vi "UHR-Fleezers Control (host) - Lorentz v4.vi"() -> ()   [LabVIEW 2014] (continued)
        n901 = case shown="True" w1439 {
          tunnel: w1436 -> [_ w1446]
          frame False {
          }
          frame True {
            n902 = local read "Time (s)"() -> (w1447:dbl)
            n903 = local read "log file ref"() -> (w1448:refnum<file>)
            n904 = call "write to event log.vi"("log file ref"=w1448, "time"=w1447, "input string"=w1446) -> ()  [unwired: 8 in]
          }
        }
        n905 = call "preamp serial write macro.vi"("String"=w1441, "Delay (ms)"=w1442, "VISA resource name"=w1445) -> ("read buffer"=→"Reply":string, "error out"=w1444:errorcluster)  [unwired: 1 out]
        n906 = call "preamp serial write macro.vi"("String"=w1441, "Delay (ms)"=w1442, "VISA resource name"=w1440) -> ()  [unwired: 3 out]
        n907 = local write "Preamp Error Out"(w1444) -> ()
      }
    }
    n908 = node-c288() -> ()  [unwired: 1 in, 1 out]
  }
  n909 = flat-sequence "Safety limits on RF frequencies and amplitudes (for AOM protection)" {
    tunnel: [w1527] -> w38
    tunnel: [w1525] -> w40
    tunnel: [w1528] -> w41
    tunnel: [w1529] -> w39
    tunnel: w22 -> [w1527]
    tunnel: T24 {"Minimum"=0.0, "Maximum"=50.0, "Increment"=1.0} ("Data Entry Limits") -> [w1525]
    tunnel: w27 -> [w1526]
    tunnel: [w1526] -> w42
    frame #0 {
      w1529 = T24 {"Minimum"=0.0, "Maximum"=40.0, "Increment"=0.1} ("Min Max Inc")
      w1528 = T24 {"Minimum"=0.0, "Maximum"=45.0, "Increment"=1.0} ("Data Entry Limits")
      n910 = property on="BD 2 Frequency 1 (MHz)" class="DigNum (strict)"("Data Range"=w1529) -> ()  [unwired: 2 in, 2 out]
      n911 = property on="BD 2 Frequency 3 (MHz)" class="DigNum (strict)"("Data Range"=w1529) -> ()  [unwired: 2 in, 2 out]
      n912 = property on="BD 2 Frequency 2 (MHz)" class="DigNum (strict)"("Data Range"=w1529) -> ()  [unwired: 2 in, 2 out]
      n913 = property on="BD 1 Frequency 1 (MHz)" class="DigNum (strict)"("Data Range"=w1527) -> ()  [unwired: 2 in, 2 out]
      n914 = property on="BD 1 Frequency 2 (MHz)" class="DigNum (strict)"("Data Range"=w1527) -> ()  [unwired: 2 in, 2 out]
      n915 = property on="BD 1 Frequency 3 (MHz)" class="DigNum (strict)"("Data Range"=w1527) -> ()  [unwired: 2 in, 2 out]
      n916 = property on="BD 2 Amplitude 1 (%)" class="DigNum (strict)"("Data Range"=w1528) -> ()  [unwired: 2 in, 2 out]
      n917 = property on="BD 2 Amplitude 2 (%)" class="DigNum (strict)"("Data Range"=w1528) -> ()  [unwired: 2 in, 2 out]
      n918 = property on="BD 2 Amplitude 3 (%)" class="DigNum (strict)"("Data Range"=w1528) -> ()  [unwired: 2 in, 2 out]
      n919 = property on="BD 1 Amplitude 3 (%)" class="DigNum (strict)"("Data Range"=w1525) -> ()  [unwired: 2 in, 2 out]
      n920 = property on="BD 1 Amplitude 2 (%)" class="DigNum (strict)"("Data Range"=w1525) -> ()  [unwired: 2 in, 2 out]
      n921 = property on="BD 1 Amplitude 1 (%)" class="DigNum (strict)"("Data Range"=w1525) -> ()  [unwired: 2 in, 2 out]
      "X RF Frequency Limits (MHz)" <- w1527
      "X RF Amplitude Limits (%)" <- w1525
      "Y RF Amplitude Limits (%)" <- w1528
      "Y RF Frequency Limits (MHz)" <- w1529
    }
  }
  n922 = stacked-sequence "Host initialization sequence - order matters!" {
    tunnel: w42 -> [_ w1549 w1641 _ w1698 w1707 w1774 w1798 _ w1841 _]
    tunnel: [_ _ _ _ _ _ _ _ _ w1841 _] -> w31
    tunnel: [_ _ _ _ _ _ _ _ _ w1840 _] -> w44
    tunnel: w41 -> [_ _ _ _ _ _ w1772 _ _ _ _]
    tunnel: w40 -> [_ _ _ _ _ _ w1771 _ _ _ _]
    tunnel: w39 -> [_ _ _ _ _ _ w1770 _ _ _ _]
    tunnel: w38 -> [_ _ _ _ _ _ w1751 _ _ _ _]
    tunnel: [_ _ _ _ _ _ _ _ w1838 _ _] -> _
    tunnel: [_ _ _ _ _ _ _ _ _ _ w1842] -> w21
    tunnel: [_ _ _ _ _ _ _ _ _ _ w1843] -> w20
    frame #0 {
    }
    frame #1 {
      w1581 = 10.0 ("y")
      w1582 = 32767.0 ("y")
      w1566 = 6.0  # clock mult.
      w1565 = 49152000.0  # TCXO frequ.
      # "Initialize some FPGA settings"
      n923 = local read "Not-Interlacing Set"() -> (w1621:enum32{"Set 1", "Set 2", "Set 3"})
      n924 = local write "Trap Pos FIFO Timeout"(u16 0 ("Trap Pos FIFO Timeout")) -> ()
      n925 = local read "Interlace"() -> (w1619:bool)
      n926 = local read "Desired Scan Incr (V)"() -> (w1593:dbl)
      n927 = local read "BD 1 Delay (ticks)"() -> (w1628:u8)
      n928 = local read "Number Interlace Sets"() -> (w1620:u8)
      n929 = local read "BD 2 Delay (Ticks)"() -> (w1629:u8)
      n930 = property on="AI Count (ticks)" class="DigNum (strict)"("Val(Sgnl)"="AI Count (ticks)") -> ()  [unwired: 2 in, 2 out]
      n931 = local read "AO1"() -> (w1587:dbl)
      n932 = local read "AO2"() -> (w1588:dbl)
      n933 = local read "Next trap write delay (ticks)"() -> (w1630:u8)
      n934 = local read "Number of scans (MCL)"() -> (w1597:u64)
      n935 = local read "Cycles/step (MCL)"() -> (w1596:u64)
      n936 = local read "Scan steps (MCL)"() -> (w1595:u64)
      n937 = local read "Continuous MCL Scanning"() -> (w1598:bool)
      n938 = Multiply(x=w1587, y=w1582) -> (x*y=w1585:dbl)
      n939 = Multiply(x=w1588, y=w1582) -> (x*y=w1583:dbl)
      n940 = Build Array("DIO count 1 (ticks)", "DIO count 2 (ticks)", "DIO count 3 (ticks)") -> (w1614:u16[])
      n941 = local read "Fast Scan Dir"() -> (w1599:bool)
      n942 = local read "2D or 1D Scan"() -> (w1611:bool)
      n943 = local read "N Acq Sets (Traps + Fl.)"() -> (w1607:i16)
      n944 = local read "Scan Increment (MHz)"() -> (w1570:dbl)
      n945 = Divide(x=w1585, y=w1581) -> (x/y=w1586:dbl)
      n946 = Divide(x=w1583, y=w1581) -> (x/y=w1584:dbl)
      n947 = To Unsigned Byte Integer(number=w1621) -> (unsigned 8bit integer=w1616:u8)
      n948 = Split 1D Array(array=w1614, index=w1620) -> (first subarray=w1612:u16[])  [unwired: 1 out]
      n949 = Multiply(x=w1593, y=32767.0) -> (x*y=w1591:dbl)
      n950 = To Word Integer(number=w1586) -> (16bit integer=w1532:i16)
      n951 = To Word Integer(number=w1584) -> (16bit integer=w1531:i16)
      n952 = Index Array(array=w1614, index=w1616) -> (element=w1615:u16)
      n953 = Add Array Elements(numeric array=w1612) -> (sum=w1613:u16)
      n954 = Multiply(x=w1565, y=w1566) -> (x*y=w1567:dbl)
      n955 = Divide(x=w1591, y=10.0) -> (x/y=w1592:dbl)
      n956 = Select(t=w1613, s=w1619, f=w1615) -> (s? t:f=w1622:u16)
      n957 = Not(x=w1599) -> (.not. x?=w1600:bool)
      n958 = To Word Integer(number=w1592) -> (16bit integer=w1594:i16)
      n959 = property on="2D or 1D Scan" class="Bool (strict)"("Val(Sgnl)"=w1611) -> ()  [unwired: 2 in, 2 out]
      n960 = Divide(x=40000000.0, y="AI Count (ticks)") -> (x/y=w1603:dbl)
      n961 = local write "Update Count (MCL)"(w1622) -> ()
      n962 = local write "Total Counts (ticks)"(w1622) -> ()
      n963 = Divide(x=w1603, y="FPGA Ave.") -> (x/y=w1602:dbl)
      n964 = local write "AI rate (Hz)"(w1603) -> ()
      n965 = Multiply(x=w1570, y=1000.0) -> (x*y=w1563:dbl)
      n966 = local write "Ave. Rate (Hz)"(w1602) -> ()
      n967 = Reciprocal(x=w1602) -> (1/x=w1601:dbl)
      n968 = Scale By Power Of 2(n=48, x=w1563) -> (x*2^n=w1562:dbl)
      n969 = local write "Ave. Period (s)"(w1601) -> ()
      n970 = Divide(x=w1562, y=w1567) -> (x/y=w1568:dbl)
      n971 = To Quad Integer(1:w1568) -> (0:w1571:i64)
      n972 = local read "Setpoints (V)"() -> (w1556:cluster{"Set 1":dbl, "Set 2":dbl})
      n973 = local read "# Samples/channel"() -> (w1578:u32)
      n974 = local read "Feedback On/Off"() -> (w1553:cluster{"Set 1":bool, "Set 2":bool})
      n975 = local read "T3 Y (V)"() -> (w1536:dbl)
      n976 = local read "T3 X (V)"() -> (w1535:dbl)
      n977 = local read "Trap intensity output range"() -> (w1546:cluster{"Normal High":i16, "Normal Low":i16})
      n978 = local read "All FB On/Off"() -> (w1552:bool)
      n979 = local read "Number of F/B Scans (AOD)"() -> (w1577:u16)
      n980 = local read "Trap Intensity PID Gains"() -> (w1545:T14)
      n981 = local read "Cycles/step (AOD)"() -> (w1573:u64)
      n982 = local read "Scan steps (AOD)"() -> (w1572:u64)
      n983 = Multiply(x=w1572, y=w1573) -> (x*y=w1574:u64)
      n984 = Multiply(x=w1574, y=u64 2) -> (x*y=w1576:u64)
      n985 = Multiply(x=w1576, y=w1577) -> (x*y=w1579:u64)
      n986 = Multiply(x=3276.7, y=w1556) -> (x*y=w1557:cluster{"Set 1":dbl, "Set 2":dbl})
      n987 = local read "Scan BD"() -> (w1561:bool)
      n988 = Multiply(x=w1536, y=32767.0) -> (x*y=w1542:dbl)
      n989 = And(x=w1553, y=w1552) -> (x .and. y?=w1554:cluster{"Set 1":bool, "Set 2":bool})
      n990 = To Word Integer(number=w1557) -> (16bit integer=w1558:cluster{"Set 1":i16, "Set 2":i16})
      n991 = Multiply(x=w1535, y=32767.0) -> (x*y=w1539:dbl)
      n992 = local read "Sets to FIFO (Traps)"() -> (w1624:T22)
      n993 = Divide(x=w1579, y=w1578) -> (x/y=w1580:dbl)
      n994 = Unbundle By Name(w1554) -> ("Set 1"=w1550:bool, "Set 2"=w1551:bool)
      n995 = Unbundle By Name(w1558) -> ("Set 1"=w1559:i16, "Set 2"=w1560:i16)
      n996 = Divide(x=w1542, y=10.0) -> (x/y=w1543:dbl)
      n997 = Divide(x=w1539, y=10.0) -> (x/y=w1538:dbl)
      n998 = To Unsigned Word Integer(number=w1543) -> (unsigned 16bit integer=w1534:u16)
      n999 = To Unsigned Word Integer(number=w1538) -> (unsigned 16bit integer=w1533:u16)
      n1000 = local read "FPGA error out"() -> (w1548:errorcluster)
      n1001 = local write "Data points/scan (f/b)"(w1576) -> ()
      n1002 = local write "Data points/scans"(w1579) -> ()
      n1003 = local write "N sets should be saved"(w1580) -> ()
      n1004 = Unbundle By Name(w1624) -> ("Set 1"=w1625:bool, "Set 2"=w1626:bool, "Set 3"=w1627:bool)
      n1005 = xnode "Read/Write Control"("FPGA VI Reference In"=w1549, "error in"=w1548, "ai count"="AI Count (ticks)", "Interlace ON/OFF"=w1619, "Number Interlace Cycles"=w1620, "Set 1"=w1625, "Set 2"=w1626, "Set 3"=w1627, "FB On/Off Set 1"=w1550, "FB On/Off Set 2"=w1551, "Interlace Off Parameters"=w1621, "FB Setpoint Set 1"=w1559, "FB Setpoint Set 2"=w1560, "Piezo Trap Y (AO4)"=w1534, "Piezo Trap X (AO5)"=w1533, "FB Gains"=w1545, "FB output range"=w1546, "Cycles per step"=w1573, "Scan BD"=w1561, "Number of scans"=w1577, "Scan steps"=w1572, "Scan freq.  increment"=w1571, "AO1"=w1532, "AO2"=w1531, "Scan freq.  increment (MCL)"=w1594, "Scan steps (MCL)"=w1595, "Cycles per step (MCL)"=w1596, "Number of scans (MCL)"=w1597, "MCL count"=w1622, "Cont. Scan (MCL)"=w1598, "MCL Scan Axis"=w1600, "1D or 2D Scan?"=w1611, "N of AI1 Int Acq Sets"=w1607, "Amp switch delay"="Amp switch delay", "Swap F1 and F2"="Swap F1 and F2", "APD to FIFO"=FALSE, "DIO count 1 (ticks)"="DIO count 1 (ticks)", "DIO count 2 (ticks)"="DIO count 2 (ticks)", "DIO count 3 (ticks)"="DIO count 3 (ticks)", "BD 1 Delay (ticks)"=w1628, "BD 2 Delay (Ticks)"=w1629, "Next trap write delay (ticks)"=w1630) -> ("error out"=w1547:errorcluster)  [unwired: 1 out]
      n1006 = local write "FPGA error out"(w1547) -> ()
    }
    frame #2 {
      # "Initialize some more FPGA settings"
      n1007 = local read "Trap Pos FB Monitor\nT1 or T2"() -> (w1652:bool)
      n1008 = local read "Trap Pos FB Negate Action"() -> (w1653:bool)
      n1009 = local read "Trap Pos. FB Offset Factor"() -> (w1654:i64)
      n1010 = local read "Trap Pos. FB Mult Factor"() -> (w1655:i64)
      n1011 = local read "Trap Pos. AI1 X Pre-scale"() -> (w1657:u16)
      n1012 = local read "Trap Pos FB Int Count"() -> (w1659:u16)
      n1013 = local read "Green Laser ON"() -> (w1631:bool)
      n1014 = local read "Neg. TTrig FPGA"() -> (w1660:bool)
      n1015 = local read "Trap Pos. FB Range"() -> (w1636:T18)
      n1016 = local read "Trap Pos. FB Gains"() -> (w1637:T17)
      n1017 = local read "Dynamic Force FB (ronen)"() -> (w1638:bool)
      n1018 = Multiply(x="Green Intensity % (FB OFF)", y=655.35) -> (x*y=w1646:dbl)
      n1019 = Multiply(x="Red FB Setpoint (mV)", y=3.2767) -> (x*y=w1668:dbl)
      n1020 = Multiply(x="Red Intensity % (FB OFF)", y=655.35) -> (x*y=w1672:dbl)
      n1021 = Unbundle By Name("Red FB Gains") -> ("proportional gain (Kc)"=w1677:i16, "integral gain (Kc*Ts/Ti)"=w1678:i16, "derivative gain (Kc*Td/Ts)"=w1679:i16)
      n1022 = Multiply(x="Green FB Setpoint (mV)", y=3.2767) -> (x*y=w1649:dbl)
      n1023 = To Unsigned Word Integer(number=w1646) -> (unsigned 16bit integer=w1648:u16)
      n1024 = To Unsigned Word Integer(number=w1672) -> (unsigned 16bit integer=w1675:u16)
      n1025 = To Word Integer(number=w1668) -> (16bit integer=w1671:i16)
      n1026 = local read "Differential FB?"() -> (w1662:bool)
      n1027 = To Word Integer(number=w1649) -> (16bit integer=w1651:i16)
      n1028 = local read "Laser interlacing mode"() -> (w1634:enum32{"Laser ON", "Laser OFF", "Interlace"})
      n1029 = local read "Invert laser interlacing"() -> (w1635:bool)
      n1030 = Unbundle By Name("Green FB Gains") -> ("proportional gain (Kc)"=w1665:i16, "integral gain (Kc*Ts/Ti)"=w1666:i16, "derivative gain (Kc*Td/Ts)"=w1667:i16)
      n1031 = Select(t=w1634, s=w1631, f=enum32{"Laser ON", "Laser OFF", "Interlace"}."Laser OFF" ("Green laser mode")) -> (s? t:f=w1633:enum32{"Laser ON", "Laser OFF", "Interlace"})
      n1032 = local read "FPGA error out"() -> (w1639:errorcluster)
      n1033 = xnode "Read/Write Control"("FPGA VI Reference In"=w1641, "error in"=w1639, "Invert GI"=w1635, "Invert GI 2"=w1635, "Invert RI"=w1635, "Invert RI 2"=w1635, "Operating Mode"=w1633, "Operating Mode 2"=w1633, "Red Laser Operating Mode"=w1633, "RI Operating Mode 2"=w1633, "P3"=w1665, "I3"=w1666, "D3"=w1667, "Green FB Setpoint"=w1651, "Green FB On/Off"="Green FB On/Off", "Current Out"=w1648, "Green int current ON count adj"="Green int current ON count adj", "Trap Pos FB Monitor T1 or T2"=w1652, "Trap Pos FB Negate Action"=w1653, "Trap Pos. FB Offset Factor"=w1654, "Trap Pos. FB Mult Factor"=w1655, "Force feedback"=FALSE, "AI1 X Scale"=w1657, "Trap Pos to FIFO"=TRUE, "Trap Pos FB Int Count"=w1659, "TTrig Negate Pos"=w1660, "FB Trig Integrate"="FB Trig Integrate", "Diff FB Measurement?"=w1662, "Negate Diff?"="Negate Diff?", "Trap pos. FB Range"=w1636, "Trap Pos. FB Gains"=w1637, "Red FB Setpoint"=w1671, "RI Current Out"=w1675, "P4"=w1677, "I4"=w1678, "D4"=w1679, "Red FB On/Off"="Red FB On/Off", "Dynamic Force FB (Ronen)"=w1638) -> ("error out"=w1640:errorcluster)  [unwired: 1 out]
      n1034 = local write "FPGA error out"(w1640) -> ()
    }
    frame #3 {
      # "Initialize more settings. Should stop using event loops to initialize."
      # "What are these?"
      n1035 = local write "Offset (nm)"(0.0 ("Offset (nm)")) -> ()
      n1036 = local write "Bead Mean (nm)"(0.0 ("Bead Mean (nm)")) -> ()
      n1037 = stacked-sequence {
        frame #0 {
          w1683 = T54."empty" ("mode")
          # "Clear external fluorescence triggering FIFO"
          # "APD loop counts"
          # "Fluorescence loop counts (rates)"
          n1038 = local read "APD Integration Time (s)"() -> (w1685:dbl)
          n1039 = local read "Interlace ON count"() -> (w1686:u16)
          n1040 = call "Smart Buffer (DBL) 1.vi"("mode"=w1683) -> ()  [unwired: 5 in, 6 out]
          n1041 = call "Smart Buffer (DBL) 2.vi"("mode"=w1683) -> ()  [unwired: 5 in, 6 out]
          n1042 = property on="APD Integration Time (s)" class="DigNum (strict)"("Val(Sgnl)"=w1685) -> ()  [unwired: 2 in, 2 out]
          n1043 = property on="Interlace ON count" class="DigNum (strict)"("Val(Sgnl)"=w1686) -> ()  [unwired: 2 in, 2 out]
          "Number of APDs" <- 3.0 ("Number of APDs")
        }
        frame #1 {
          # "Number of APDs affects\nAPD DMA transfer"
          # "General settings for all lasers:"
          # "And includes all laser\nON/OFF settings"
          # "Fluorescent lasers settings:"
          # "Blue laser settings:"
          n1044 = local read "Laser interlacing mode"() -> (w1688:enum32{"Laser ON", "Laser OFF", "Interlace"})
          n1045 = local read "Invert laser interlacing"() -> (w1687:bool)
          n1046 = local read "Blue FB On/Off"() -> (w1689:bool)
          n1047 = property on="Blue FB On/Off" class="Bool (strict)"("Val(Sgnl)"=w1689) -> ()  [unwired: 2 in, 2 out]
          n1048 = property on="Invert laser interlacing" class="Bool (strict)"("Val(Sgnl)"=w1687) -> ()  [unwired: 2 in, 2 out]
          n1049 = property on="Laser interlacing mode" class="RadioBtnsControl (strict)"("Val(Sgnl)"=w1688) -> ()  [unwired: 2 in, 2 out]
        }
        frame #2 {
          w1690 = path "C:/Home/Bustamante Lab/Comstock-LabView-Link.udl" ("connection information")
          # "Database link changed by Ronen - not clear if it matter for the program."
          # "Initialize the database connection"
          n1050 = disable-structure shown="Disabled" {
            disable-tunnel: [w1693 _] -> w1691
            disable-tunnel: w1690 -> [w1692 _]
            frame Disabled {
              n1051 = call-poly <vilib>:"DB Tools Open Connection.vi"("connection information"=w1692) -> ("connection reference"=w1693:T25)  [unwired: 7 in, 1 out]
            }
            frame Enabled {
            }
          }
          "connection reference" <- w1691
          n1052 = local write "connection reference"(w1691) -> ()
          n1053 = local write "Database link"(w1690) -> ()
        }
        frame #3 {
          # "Load active calibration to fpga"
          n1054 = local read "Base N trap periods"() -> (w1695:u32)
          n1055 = local read "T1 Osc Enable"() -> (w1694:bool)
          n1056 = property on="T1 Osc Enable" class="Bool (strict)"("Val(Sgnl)"=w1694) -> ()  [unwired: 2 in, 2 out]
          n1057 = property on="Base N trap periods" class="DigNum (strict)"("Val(Sgnl)"=w1695) -> ()  [unwired: 2 in, 2 out]
        }
      }
    }
    frame #4 {
      # "Set FIFO size and run FPGA"
      n1058 = local read "FPGA error out"() -> (w1697:errorcluster)
      n1059 = xnode "Invoke Method"("FPGA VI Reference In"=w1698, "error in"=w1697, "Requested Depth"="Trap AI FIFO Depth") -> ("FPGA VI Reference Out"=w1702:T50, "error out"=w1703:errorcluster)  [unwired: 1 out]
      n1060 = xnode "Invoke Method"("FPGA VI Reference In"=w1702, "error in"=w1703, "Requested Depth"="Trap Position FIFO Depth") -> ("FPGA VI Reference Out"=w1700:T50, "error out"=w1699:errorcluster)  [unwired: 1 out]
      n1061 = xnode "Invoke Method"("FPGA VI Reference In"=w1700, "error in"=w1699) -> ("error out"=w1696:errorcluster)  [unwired: 1 in, 1 out]
      n1062 = local write "FPGA error out"(w1696) -> ()
    }
    frame #5 {
      # "Adjust FPGA timing loop phases"
      n1063 = flat-sequence "Initial FPGA Loop Relative Phase Adjustment" {
        tunnel: "Initial Phase Adjustment (AI1)" -> [w1737]
        tunnel: "Initial Phase Adjustment (GI)" -> [w1736]
        tunnel: "Initial Phase Adj. (MCL)" -> [w1735]
        tunnel: [w1738] -> w1722
        tunnel: [w1734] -> w1721
        tunnel: "Initial Phase Adjustment (APD Acq)" -> [w1733]
        tunnel: "Initial Phase Adjustment (APD 1 Gate)" -> [w1732]
        tunnel: "Initial Phase Adjustment (Green FB)" -> [w1731]
        tunnel: "Initial Phase Adjustment (GI) 2" -> [w1730]
        tunnel: "Initial Phase Adjustment (APD 2 Gate)" -> [w1729]
        tunnel: "Initial Phase Adjustment (RI)" -> [w1728]
        tunnel: "Initial Phase Adjustment (BI DO)" -> [w1727]
        tunnel: "Initial Phase Adjustment (BI AO)" -> [w1726]
        tunnel: "Initial Phase Adjustment (APD 3 Gate)" -> [w1725]
        tunnel: w1707 -> [w1724]
        tunnel: w1722 -> [w1740]
        tunnel: [w1741] -> w1720
        tunnel: w1721 -> [w1741]
        tunnel: [w1740] -> w1719
        tunnel: w1720 -> [w1745]
        tunnel: w1719 -> [w1744]
        tunnel: [w1742] -> w1706
        frame #0 {
          n1064 = local read "FPGA error out"() -> (w1723:errorcluster)
          n1065 = xnode "Read/Write Control"("FPGA VI Reference In"=w1724, "error in"=w1723, "Phase count adjustment"=w1737, "Phase count adjustment (GI)"=w1736, "Phase count adjustment (MCL)"=w1735, "Phase Count Adjustment (APD Acq)"=w1733, "Phase count adjustment (APD 1 Gate)"=w1732, "Phase count adjustment (APD 2 Gate)"=w1729, "Phase count adjustment (Green FB)"=w1731, "Phase count adjustment (GI) 2"=w1730, "Phase count adjustment (RI)"=w1728, "Phase count adjustment (BI AO)"=w1726, "Phase count adjustment (BI D)"=w1727, "Phase count adjustment (APD 3 Gate)"=w1725) -> ("FPGA VI Reference Out"=w1734:T50, "error out"=w1738:errorcluster)
        }
        frame #1 {
          n1066 = Wait (ms)(milliseconds to wait=u32 100) -> ()  [unwired: 1 out]
        }
        frame #2 {
          w1743 = TRUE
          n1067 = xnode "Read/Write Control"("FPGA VI Reference In"=w1745, "error in"=w1744, "+ phase"=w1743, "+ phase (GI)"=w1743, "+ phase (MCL)"=w1743, "+ phase (APD Acq)"=w1743, "+ phase (APD 1 Gate)"=w1743, "+ phase (APD 2 Gate)"=w1743, "+ phase (Green FB)"=w1743, "+ phase (GI) 2"=w1743, "+ phase (RI)"=w1743, "+ phase (BI AO)"=w1743, "+ phase (BI D)"=w1743, "+ phase (APD 3 Gate)"=w1743) -> ("error out"=w1742:errorcluster)  [unwired: 1 out]
        }
      }
      n1068 = local write "FPGA error out"(w1706) -> ()
    }
    frame #6 {
      w1759 = 6.0  # clock mult.
      w1758 = 49152000.0  # TCXO frequ.
      w1763 = 6.0  # clock mult.
      w1764 = 49152000.0  # TCXO frequ.
      # "Added by ronen - definition of \nlimit frequencies when using dynamic feedback"
      # "Initialize trap RF synth board and set initial frequencies and amplitudes"
      n1069 = local read "FPGA error out"() -> (w1773:errorcluster)
      n1070 = call "Initialize RF boards - interlace 3.vi"("error in"=w1773, "FPGA VI Reference In"=w1774) -> ("error out"=w1775:errorcluster, "FPGA VI Reference Out"=w1795:T50)
      n1071 = call "set RF board frequency - interlace.vi"("Board 2 Frequency Limits"=w1770, "Board 1 Frequency Limits"=w1751, "error in"=w1775, "FPGA VI Reference In"=w1795, "Board 2 Frequency 3 (MHz)"="BD 2 Frequency 3 (MHz)", "Board 1 Frequency 3 (MHz)"="BD 1 Frequency 3 (MHz)", "Board 2 Frequency 2 (MHz)"="BD 2 Frequency 2 (MHz)", "Board 2 Frequency 1 (MHz)"="BD 2 Frequency 1 (MHz)", "Board 1 Frequency 2 (MHz)"="BD 1 Frequency 2 (MHz)", "Board 1 Frequency 1  (MHz)"="BD 1 Frequency 1 (MHz)") -> ("error out"=w1778:errorcluster, "FPGA VI Reference Out"=w1750:T50)
      n1072 = Unbundle By Name(w1751) -> ("Maximum"=w1761:dbl, "Minimum"=w1752:dbl)
      n1073 = call "set RF board amplitude - interlace.vi"("Board 2 Amplitude Limits"=w1772, "Board 1 Amplitude Limits"=w1771, "error in"=w1778, "FPGA VI Reference In"=w1750, "Board 2 Amplitude 3 (%)"="BD 2 Amplitude 3 (%)", "Board 1 Amplitude 3 (%)"="BD 1 Amplitude 3 (%)", "Board 2 Amplitude 2 (%)"="BD 2 Amplitude 2 (%)", "Board 2 Amplitude 1 (%)"="BD 2 Amplitude 1 (%)", "Board 1 Amplitude 2 (%)"="BD 1 Amplitude 2 (%)", "Board 1 Amplitude 1 (%)"="BD 1 Amplitude 1 (%)") -> ("error out"=w1747:errorcluster)  [unwired: 1 out]
      n1074 = Multiply(x=w1752, y=1000000.0) -> (x*y=w1756:dbl)
      n1075 = Multiply(x=w1761, y=1000000.0) -> (x*y=w1766:dbl)
      n1076 = Scale By Power Of 2(n=48, x=w1756) -> (x*2^n=w1754:dbl)
      n1077 = Subtract(x="BD 1 Frequency 1 (MHz)", y="BD 1 Frequency 2 (MHz)") -> (x-y=w1785:dbl)
      n1078 = Subtract(x="BD 2 Frequency 1 (MHz)", y="BD 2 Frequency 2 (MHz)") -> (x-y=w1786:dbl)
      n1079 = Scale By Power Of 2(n=48, x=w1766) -> (x*2^n=w1768:dbl)
      n1080 = Multiply(x=w1758, y=w1759) -> (x*y=w1760:dbl)
      n1081 = Multiply(x=w1764, y=w1763) -> (x*y=w1762:dbl)
      n1082 = Square(x=w1786) -> (x^2=w1788:dbl)
      n1083 = Square(x=w1785) -> (x^2=w1787:dbl)
      n1084 = Divide(x=w1754, y=w1760) -> (x/y=w1755:dbl)
      n1085 = Divide(x=w1768, y=w1762) -> (x/y=w1767:dbl)
      n1086 = Add(x=w1787, y=w1788) -> (x+y=w1789:dbl)
      n1087 = To Unsigned Quad Integer(1:w1755) -> (0:w1748:u64)
      n1088 = To Unsigned Quad Integer(1:w1767) -> (0:w1749:u64)
      n1089 = Square Root(x=w1789) -> (sqrt(x)=w1790:dbl)
      n1090 = local write "Trap Delta (MHz)"(w1790) -> ()
      n1091 = xnode "Read/Write Control"("FPGA VI Reference In"=w1750, "error in"=w1747, "FB Max Frequency"=w1749, "FB Min frequency"=w1748) -> ("error out"=w1746:errorcluster)  [unwired: 1 out]
      n1092 = local write "FPGA error out"(w1746) -> ()
    }
    frame #7 {
      n1093 = local read "FPGA error out"() -> (w1797:errorcluster)
      n1094 = flat-sequence {
        tunnel: [w1811] -> w1802
        tunnel: [w1810] -> w1801
        tunnel: w1798 -> [w1804]
        tunnel: w1797 -> [w1803]
        tunnel: [w1815] -> w1800
        tunnel: w1802 -> [w1815]
        tunnel: [w1814] -> w1799
        tunnel: w1801 -> [w1814]
        tunnel: w1800 -> [w1823]
        tunnel: w1799 -> [w1822]
        tunnel: [w1817] -> w1796
        frame #0 {
          n1095 = xnode "Read/Write Control"("FPGA VI Reference In"=w1804, "error in"=w1803, "Direct RF Box  Communication"=FALSE) -> ("FPGA VI Reference Out"=w1811:T50, "error out"=w1810:errorcluster)
          n1096 = local read "Trap 1 (ON/OFF)"() -> (w1805:bool)
          n1097 = local write "Saving..."(FALSE ("Saving Data")) -> ()
          n1098 = local write "Stop All"(FALSE ("Stop All")) -> ()
          n1099 = local write "Index"(1.0 ("Index")) -> ()
          n1100 = property on="Trap 1 ON" class="Bool (strict)"("Value"=w1805) -> ()  [unwired: 2 in, 2 out]
          "Manipulating Trap" <- FALSE ("Manipulating Trap")
        }
        frame #1 {
          n1101 = local read "Trap 2 (ON/OFF)"() -> (w1813:bool)
          n1102 = Wait (ms)(milliseconds to wait=u32 10) -> ()  [unwired: 1 out]
          n1103 = property on="Trap 2 ON" class="Bool (strict)"("Val(Sgnl)"=w1813) -> ()  [unwired: 2 in, 2 out]
        }
        frame #2 {
          n1104 = local read "Scan Range (nm)"() -> (w1818:dbl)
          n1105 = xnode "Read/Write Control"("FPGA VI Reference In"=w1823, "error in"=w1822, "FPGA Controls  RF Box"=TRUE ("Direct RF Box  Communication")) -> ("error out"=w1817:errorcluster)  [unwired: 1 out]
          n1106 = call "Update messages.vi"("Message to add"="UHR-Fleezers ready.", "Old message string"="") -> ("New message string"=w1821:string)
          n1107 = local write "Messages"(w1821) -> ()
          n1108 = property on="Scan Range (nm)" class="DigNum (strict)"("Val(Sgnl)"=w1818) -> ()  [unwired: 2 in, 2 out]
        }
      }
      n1109 = local write "FPGA error out"(w1796) -> ()
    }
    frame #8 {
      w1830 = u32 0
      w1836 = cluster{u32, u32} {16777238, 16777238}
      w1831 = 0.0
      n1110 = control-ref of="Piezo trap cursor control"() -> (w1832:refnum<vi>)
      n1111 = property class="XYGraph (strict)"(reference=w1832, "XScale.Maximum"=10.0, "XScale.Minimum"=w1831, "YScale.Maximum"=w1831, "YScale.Minimum"=-10.0, "Plot Area Colors"=w1836, "Frame Color"=u32 9868950, "XScale.GridColors"=w1836, "YScale.GridColors"=w1836, "Cursor.Cursor Color"=u32 16711680, "Active Cursor"=w1830, "Cursor.CursorMode"=w1830) -> ()  [unwired: 1 in, 2 out]
      n1112 = call "hamilton_controller.vi"("VISA resource name in"="Visa resource for valves", "action"=T53."CONNECT") -> ("error out"=w1829:errorcluster, "VISA resource name out"=w1826:refnum<visa-resource-name>)  [unwired: 8 in]
      n1113 = call "hamilton_controller.vi"("VISA resource name in"=w1826, "error in"=w1829, "action"=T53."INITIALIZE VALVES") -> ("error out"=w1838:errorcluster)  [unwired: 7 in, 1 out]
    }
    frame #9 {
      # "Wait 5 s for all the event loops still being executed to finish."
      n1114 = Wait (ms)(milliseconds to wait=u32 5000) -> ()  [unwired: 1 out]
      n1115 = local read "FPGA error out"() -> (w1840:errorcluster)
    }
    frame #10 {
      # "Initialize Serial communication with Arduino, and clear the buffer first"
      n1116 = Unbundle By Name("Serial Settings for arduino") -> ("baud rate"=w1855:u32, "data bits"=w1854:u16, "parity"=w1853:enum16{"None", "Odd", "Even", "Mark", "Space"}, "stop bits"=w1852:u16, "flow control"=w1851:u16, "Time out (ms)"=w1849:u32)
      n1117 = call-poly "VISA Configure Serial Port"("VISA resource name"="VISA resource name", "timeout (10sec)"=w1849, "Enable Termination\nChar (T)"=FALSE, "baud rate (9600)"=w1855, "data bits (8)"=w1854, "parity (0:none)"=w1853, "error in (no error)"="Serial Error in", "stop bits (10: 1 bit)"=w1852, "flow control (0:none)"=w1851) -> ("VISA resource name out"=w1845:refnum<visa-resource-name>, "error out"=w1844:errorcluster)  [unwired: 5 in]
      n1118 = VISA Clear(VISA resource name=w1845, error in (no error)=w1844) -> (VISA resource name out=w1842:refnum<visa-resource-name>, error out=w1843:errorcluster)
    }
  }
  n1119 = node-c288() -> (w51:T35)  [unwired: 4 out]
  n1120 = disable-structure shown="Disabled" {
    frame Disabled {
      n1121 = while "Duncan's play event loop" {
        stop <- w1858 stop-if-true
        n1122 = Create User Event(user event datatype=TRUE ("Boolean")) -> (user event=w1859:refnum<user-event>)  [unwired: 1 in, 1 out]
        n1123 = Create User Event(user event datatype=TRUE ("Boolean")) -> (user event=w1865:refnum<user-event>)  [unwired: 1 in, 1 out]
        n1124 = global write "Global for fluorescence simulation mean (30 samples), (power series).vi" "Red Signal"(w1859) -> ()
        n1125 = global write "Global for fluorescence simulation mean (30 samples), (power series).vi" "Green Signal"(w1865) -> ()
        n1126 = register-events(w1865, w1859) -> (reference out=w1864:refnum<event-registration>)  [unwired: 2 in, 1 out]
        n1127 = event shown="[1] \"Start assembly line\": Value Change" {
          selector: w1864 -> [_ _ _ _]
          dyn-events: _ -> [_ _ _ _]
          timeout: 100 -> [_ _ _ _]
          event Timeout {
            n1128 = event-data() -> ()  [unwired: 1 in, 2 out]
          }
          event "Start assembly line": Value Change {
            n1129 = event-data() -> ("OldVal"=w1867:bool)  [unwired: 1 in, 4 out]
            n1130 = case shown="True" w1867 {
              selector: w1867 -> [_ w1868]
              frame False {
              }
              frame True {
                n1131 = property on="Move to Position 3" class="Bool"("Val(Sgnl)"=w1868) -> ()  [unwired: 2 in, 2 out]
                n1132 = case shown="1" "Numeric" {
                  frame 0, Default {
                  }
                  frame 1 {
                    n1133 = property on="Green Laser ON" class="Bool (strict)"("Val(Sgnl)"=TRUE ("Value (Signaling)")) -> ()  [unwired: 2 in, 2 out]
                  }
                  frame 2 {
                    n1134 = property on="Red Laser ON" class="Bool (strict)"("Val(Sgnl)"=TRUE) -> ()  [unwired: 2 in, 2 out]
                  }
                }
              }
            }
          }
          event User Event {
            n1135 = event-data() -> ("Boolean"=w1872:bool)  [unwired: 1 in, 3 out]
            "Green Fluorophore" <- w1872
            n1136 = property on="Start assembly line" class="Bool"("Val(Sgnl)"=w1872) -> ()  [unwired: 2 in, 2 out]
          }
          event User Event {
            n1137 = event-data() -> ("Boolean"=w1873:bool)  [unwired: 1 in, 3 out]
            "Red Fluorophore" <- w1873
            n1138 = property on="Start assembly line" class="Bool"("Val(Sgnl)"=w1873) -> ()  [unwired: 2 in, 2 out]
          }
        }
        n1139 = property on="Get Fluorophore" class="Bool (strict)"("Val(Sgnl)"="Get Fluorophore") -> ()  [unwired: 2 in, 2 out]
        n1140 = Wait (ms)(milliseconds to wait=u32 100) -> ()  [unwired: 1 out]
        n1141 = local read "Stop All"() -> (w1857:bool)
        n1142 = Or(x=w1857, y="stop") -> (x .or. y?=w1858:bool)
      }
    }
    frame Enabled {
    }
  }
  n1143 = timed-loop "Rough control of MCL mirror stage (debugging)" {
    tunnel: [w1876] -> w92
    timing: w51 -> [_]
    timing-out: [_] -> w50
    tunnel: w42 -> [w1874]
    stop <- w1876 stop-if-true
    n1144 = node-c288() -> ()  [unwired: 2 out]
    n1145 = case shown="1" "MCL Mode" {
      tunnel: w1874 -> [_ w1879 w1926]
      frame 0, Default {
      }
      frame 1 {
        n1146 = node-c288() -> (w1881:T35)  [unwired: 4 out]
        n1147 = timed-loop "Oscillate MCL mirror" {
          timing: w1881 -> [_]
          timing-out: [_] -> w1880
          tunnel: w1879 -> [w1882]
          i -> [w1920]
          stop <- w1883 stop-if-true
          n1148 = node-c288() -> (w1919:i64)  [unwired: 1 out]
          n1149 = Multiply(x="AO1", y=32767.0) -> (x*y=w1915:dbl)
          n1150 = Multiply(x="AO2", y=32767.0) -> (x*y=w1910:dbl)
          n1151 = Divide(x=w1915, y=10.0) -> (x/y=w1916:dbl)
          n1152 = Divide(x=w1910, y=10.0) -> (x/y=w1911:dbl)
          n1153 = To Word Integer(number=w1916) -> (16bit integer=w1908:i16)
          n1154 = To Word Integer(number=w1911) -> (16bit integer=w1907:i16)
          n1155 = Divide(x=w1919, y=i64 1000) -> (x/y=w1890:dbl)
          n1156 = Multiply(x=w1890, y=w1920) -> (x*y=w1901:dbl)
          n1157 = Multiply(x="Osc. freq. (Hz) 2", y=6.283185307179586) -> (x*y=w1902:dbl)
          n1158 = Multiply(x=w1902, y=w1901) -> (x*y=w1900:dbl)
          n1159 = Sine(x=w1900) -> (sin(x)=w1899:dbl)
          n1160 = Multiply(x=w1899, y="Osc. amp. (V)") -> (x*y=w1897:dbl)
          n1161 = Add(x=w1897, y="Osc. center (V)") -> (x+y=w1895:dbl)
          n1162 = Divide(x=w1895, y=10.0) -> (x/y=w1893:dbl)
          n1163 = Multiply(x=w1893, y=32767.0) -> (x*y=w1888:dbl)
          n1164 = Select(t=w1888, s="Scan axis", f=w1908) -> (s? t:f=w1906:dbl)
          n1165 = Select(t=w1907, s="Scan axis", f=w1888) -> (s? t:f=w1905:dbl)
          n1166 = local read "MCL Mode"() -> (w1887:u16)
          n1167 = Not Equal?(x=w1887, y=u16 1) -> (x != y?=w1884:bool)
          n1168 = local read "Stop All"() -> (w1885:bool)
          n1169 = xnode "Read/Write Control"("FPGA VI Reference In"=w1882, "AO1"=w1906, "AO2"=w1905) -> ()  [unwired: 1 in, 2 out]
          n1170 = Compound Arithmetic op=OR(w1885, w1884) -> (w1883:bool)
          n1171 = node-c288() -> ()  [unwired: 2 out]
        }
        n1172 = node-c288(w1880) -> ()  [unwired: 1 out]
      }
      frame 2 {
        n1173 = case shown="True" "Start Scan" {
          tunnel: w1926 -> [_ w1928]
          frame False {
          }
          frame True {
            n1174 = Subtract(x="End (V)", y="Begin (V)") -> (x-y=w1935:dbl)
            n1175 = Decrement(x="N Points") -> (x-1=w1934:dbl)
            n1176 = Divide(x=w1935, y=w1934) -> (x/y=w1932:dbl)
            n1177 = for {
              N: "N Points" -> [_]
              tunnel: "Begin (V)" -> [w1951]
              tunnel: [w1943] -> w1938 mode=indexing
              tunnel: w1932 -> [w1942]
              tunnel: [w1940] -> w1931 mode=indexing
              tunnel: w1928 -> [w1939]
              i -> [w1950]
              n1178 = Multiply(x=w1942, y=w1950) -> (x*y=w1949:dbl)
              n1179 = Add(x=w1951, y=w1949) -> (x+y=w1946:dbl)
              n1180 = local read "Scan axis"() -> (w1941:bool)
              n1181 = local read "AO1"() -> (w1948:dbl)
              n1182 = local read "AO2"() -> (w1947:dbl)
              n1183 = Select(t=w1946, s=w1941, f=w1948) -> (s? t:f=w1945:dbl)
              n1184 = Select(t=w1947, s=w1941, f=w1946) -> (s? t:f=w1944:dbl)
              n1185 = flat-sequence {
                tunnel: w1945 -> [w1955]
                tunnel: w1944 -> [w1954]
                tunnel: w1939 -> [w1952]
                tunnel: [w1965] -> w1943
                tunnel: [w1964] -> w1940
                frame #0 {
                  w1958 = 10.0 ("y")
                  w1953 = 32767.0 ("y")
                  n1186 = Multiply(x=w1955, y=w1953) -> (x*y=w1961:dbl)
                  n1187 = Multiply(x=w1954, y=w1953) -> (x*y=w1959:dbl)
                  n1188 = Divide(x=w1961, y=w1958) -> (x/y=w1962:dbl)
                  n1189 = Divide(x=w1959, y=w1958) -> (x/y=w1960:dbl)
                  n1190 = To Word Integer(number=w1962) -> (16bit integer=w1956:i16)
                  n1191 = To Word Integer(number=w1960) -> (16bit integer=w1957:i16)
                  n1192 = xnode "Read/Write Control"("FPGA VI Reference In"=w1952, "AO1"=w1956, "AO2"=w1957) -> ()  [unwired: 1 in, 2 out]
                }
                frame #1 {
                  n1193 = Wait (ms)(milliseconds to wait="DAQ Delay (ms)") -> ()  [unwired: 1 out]
                }
                frame #2 {
                  n1194 = local read "Slow mean"() -> (w1965:dbl)
                  n1195 = local read "Sigma"() -> (w1964:dbl)
                }
              }
            }
            n1196 = Bundle("Begin (V)"="Begin (V)", w1932, w1938) -> (→"MCL Scan":cluster{"Begin (V)":dbl, dbl, dbl[]})  [unwired: 1 out]
            n1197 = Bundle("Begin (V)"="Begin (V)", w1932, w1931) -> (→"MCL Scan 2":cluster{"Begin (V)":dbl, dbl, dbl[]})  [unwired: 1 out]
          }
        }
      }
    }
    n1198 = local read "Stop All"() -> (w1876:bool)
    n1199 = node-c288() -> ()  [unwired: 2 out]
  }
  n1200 = node-c288(2 ("Processor")) -> (w83:T35)  [unwired: 3 out]
  n1201 = timed-loop "Basic control parameters (all FPGA settings, other basic controls)" {
    shift-right: [w1973] -> _
    shift-left: errorcluster {"status"=FALSE, "code"=0, "source"=""} ("error out") -> [_]
    tunnel: [w1972] -> _
    timing: w83 -> [_]
    timing-out: [_] -> w82
    tunnel: w64 -> [w1971]
    tunnel: w60 -> [w1970]
    tunnel: w59 -> [w1969]
    tunnel: w58 -> [w1968]
    tunnel: w57 -> [w1967]
    tunnel: w42 -> [w1966]
    stop <- w1972 stop-if-true
    n1202 = node-c288() -> ()  [unwired: 2 out]
    n1203 = event shown="[0] \"AI Count (ticks)\", \"Sets to FIFO (Traps)\", \"Save ave N\", \"FPGA Ave.\", \"# Samples/channel\", \"N sets to save\": Value Change" {
      selector: _ -> [_ _ _ _ _ _ _ _ _ _ _ _ _ _ _ _ _ _ _ _ _ _ _ _ _ _ _ _ _ _ _ _ _ _ _ _ _ _ _ _ _ _ _ _ _ _ _ _ _ _ _ _ _ _ _ _ _ _ _ _ _ _ _ _ _ _ _ _ _ _ _ _ _ _ _ _ _ _ _ _ _ _ _ _ _ _]
      dyn-events: _ -> [_ _ _ _ _ _ _ _ _ _ _ _ _ _ _ _ _ _ _ _ _ _ _ _ _ _ _ _ _ _ _ _ _ _ _ _ _ _ _ _ _ _ _ _ _ _ _ _ _ _ _ _ _ _ _ _ _ _ _ _ _ _ _ _ _ _ _ _ _ _ _ _ _ _ _ _ _ _ _ _ _ _ _ _ _ _]
      timeout: _ -> [_ _ _ _ _ _ _ _ _ _ _ _ _ _ _ _ _ _ _ _ _ _ _ _ _ _ _ _ _ _ _ _ _ _ _ _ _ _ _ _ _ _ _ _ _ _ _ _ _ _ _ _ _ _ _ _ _ _ _ _ _ _ _ _ _ _ _ _ _ _ _ _ _ _ _ _ _ _ _ _ _ _ _ _ _ _]
      tunnel: [w2013 _ _ _ w2040 _ _ _ _ _ _ _ w2146 _ _ w2233 w2235 w2242 w2244 w2314 _ w2356 w2382 w2410 w2435 w2462 w2488 w2517 _ w2522 w2616 w2620 w2657 _ w2720 w2723 w2726 w2736 w2739 _ w2746 _ _ _ _ _ _ _ _ _ _ _ _ _ _ _ _ _ _ _ w3241 _ _ _ _ w3278 _ _ _ _ _ _ _ _ _ _ _ _ _ _ _ _ _ _ _ _] -> w1973
      tunnel: [_ _ _ _ _ _ _ _ _ _ w2125 _ _ _ _ _ _ _ _ _ _ _ _ _ _ _ _ _ _ _ _ _ _ _ _ _ _ _ _ _ _ _ _ _ _ _ _ _ _ _ _ _ _ _ _ _ _ _ _ _ _ _ _ _ _ _ _ _ _ _ _ _ _ _ _ _ _ _ _ _ _ _ _ _ _ _] -> w1972
      tunnel: [_ _ _ _ _ _ _ _ "Round T1 X" _ _ _ _ _ _ _ _ _ _ _ _ _ _ _ _ _ _ _ _ _ _ _ _ _ _ _ _ _ _ _ _ _ _ _ _ _ _ _ _ _ _ _ _ _ _ _ _ _ _ _ _ _ _ _ _ _ _ _ _ _ _ _ _ _ _ _ _ _ _ _ _ _ _ _ _ _] -> _
      tunnel: [_ _ _ "Adjust Scale\nto Mean" _ _ _ _ _ _ _ _ _ _ _ _ _ _ _ _ _ _ _ _ _ _ _ _ _ "Test ttrig" _ _ _ _ _ _ _ _ _ _ _ _ _ _ _ _ _ _ _ _ w2988 w3052 w3099 w3148 _ _ _ _ _ _ _ _ _ _ _ _ _ _ _ _ _ _ _ _ _ _ _ _ _ _ _ _ _ _ _ _] -> _
      tunnel: [_ _ _ _ _ _ _ _ _ "Round T2 X" _ "Delayed Interlace Start" _ _ _ _ _ _ _ _ _ _ _ _ _ _ _ _ _ _ _ _ _ _ _ _ _ _ _ _ _ _ _ _ _ _ _ _ _ _ _ _ _ _ _ _ _ _ _ _ _ _ _ _ _ _ _ _ _ _ _ _ _ _ _ _ _ _ _ _ _ _ _ _ _ _] -> _
      tunnel: w1971 -> [_ _ _ _ _ _ _ _ _ _ _ _ _ _ _ _ _ _ _ _ _ _ _ _ _ _ _ _ _ _ _ _ _ _ _ _ _ _ _ _ _ _ _ _ _ _ w2958 w2966 w2973 w2979 w2987 _ _ w3147 _ _ _ _ _ _ _ _ _ _ _ _ _ _ _ _ _ _ _ _ _ _ _ _ _ _ _ _ _ _ _ _]
      tunnel: w1970 -> [_ _ _ _ _ _ _ _ _ _ _ _ _ _ _ _ _ _ _ _ _ _ _ _ _ _ _ _ _ _ _ _ _ _ _ _ _ _ _ _ _ _ _ _ w2845 _ _ _ _ _ _ w3051 _ _ w3154 _ w3166 _ w3182 _ _ _ _ _ _ _ _ _ _ _ _ _ _ _ _ _ _ _ _ _ _ _ _ _ _ _]
      tunnel: w1969 -> [_ _ _ _ _ _ _ _ _ _ _ _ _ _ _ _ _ _ _ _ _ _ _ _ _ _ _ _ _ _ _ _ _ _ _ _ _ _ _ _ _ _ _ _ _ _ _ _ _ _ _ _ _ _ _ _ _ _ _ _ _ _ _ _ _ _ _ _ _ _ _ _ _ _ _ _ _ _ _ _ _ _ _ _ _ _]
      tunnel: w1968 -> [_ _ _ _ _ _ _ _ _ _ _ _ _ _ _ _ _ _ _ _ _ _ _ _ _ _ _ _ _ _ _ _ _ _ _ _ _ _ _ _ _ w2757 _ _ _ _ _ _ _ _ _ _ w3098 _ _ w3160 _ w3174 _ w3208 _ _ _ _ _ _ _ _ _ _ _ _ _ _ _ _ _ _ _ _ _ _ _ _ _ _]
      tunnel: w1967 -> [_ _ _ _ _ _ _ _ _ _ _ _ _ _ _ _ _ _ _ _ _ _ _ _ _ _ _ _ _ _ _ _ _ _ _ _ _ _ _ _ _ _ _ _ _ _ _ _ _ _ _ _ _ _ _ _ _ _ _ _ _ _ _ _ _ _ _ _ _ _ _ _ _ _ _ _ _ _ _ _ _ _ _ _ _ _]
      tunnel: w1966 -> [w1976 _ _ _ w2039 _ w2065 _ _ _ _ _ w2137 _ _ w2217 w2234 w2241 w2243 w2279 _ w2345 w2380 w2392 w2417 w2445 w2465 w2493 w2518 w2520 w2524 w2617 w2621 _ w2717 w2721 w2724 w2734 w2737 _ w2745 _ _ _ _ _ _ _ _ _ _ _ _ _ _ _ _ _ _ _ w3234 _ w3255 _ w3262 w3277 _ w3284 w3311 w3318 w3334 w3342 _ w3353 _ w3397 _ _ w3451 w3482 w3486 w3494 _ w3558 w3568 w3587]
      tunnel: [_ _ _ _ _ _ _ _ _ _ w2124 _ _ _ _ _ _ _ _ _ _ _ _ _ _ _ _ _ _ _ _ _ _ _ _ _ _ _ _ _ _ _ w2837 w2841 _ _ _ _ _ _ _ _ _ _ _ _ _ _ _ _ _ _ _ _ _ _ _ _ _ _ _ _ _ _ _ _ _ _ _ _ _ _ _ _ _ _] -> _
      event "AI Count (ticks)", "Sets to FIFO (Traps)", "Save ave N", "FPGA Ave.", "# Samples/channel", "N sets to save": Value Change {
        # "RG 18-01-16 Increased amount of elements to read for trap position, to add x and y for piezo trap"
        # "So that if 'Save ave N' is updated, the AOD scanning code updates too."
        n1204 = event-data() -> ()  [unwired: 6 out]
        n1205 = local read "AI Count (ticks)"() -> (w1997:u16)
        n1206 = Divide(x=40000000.0, y=w1997) -> (x/y=w1989:dbl)
        "AI rate (Hz)" <- w1989
        "Ave. Rate (Hz)" <- w1989
        n1207 = Reciprocal(x=w1989) -> (1/x=→"Ave. Period (s)":dbl)
        n1208 = Unbundle By Name("Sets to FIFO (Traps)") -> ("Set 1"=w1980:bool, "Set 2"=w1979:bool, "Set 3"=w1978:bool)
        n1209 = Divide(x=w1989, y="N Acq Sets (Traps + Fl.)") -> (x/y=w2010:dbl)
        "Data Rate (Hz)" <- w2010
        n1210 = Reciprocal(x=w2010) -> (1/x=→"Data Period (s)":dbl)
        n1211 = Boolean To (0,1)(Boolean="Sets to FIFO (Traps)") -> (0, 1=w2005:cluster{"Set 1":i16, "Set 2":i16, "Set 3":i16})
        n1212 = xnode "Read/Write Control"("FPGA VI Reference In"=w1976, "ai count"=w1997, "Set 1"=w1980, "Set 2"=w1979, "Set 3"=w1978, "N of AI1 Int Acq Sets"="N Acq Sets (Traps + Fl.)") -> ("error out"=w2013:errorcluster)  [unwired: 1 in, 1 out]
        n1213 = Cluster To Array(cluster=w2005) -> (array=w2004:i16[])
        n1214 = local read "Save ave N"() -> (w2009:dbl)
        n1215 = To Unsigned Long Integer(number=w2004) -> (unsigned 32bit integer=w1986:u32[])
        n1216 = local read "Scan steps (AOD)"() -> (w2006:u64)
        n1217 = Multiply(x=w1997, y="N Acq Sets (Traps + Fl.)") -> (x*y=w1995:u16)
        n1218 = Add Array Elements(numeric array=w1986) -> (sum=w1998:u32)
        "Trap Sets" <- w1998
        n1219 = Divide(x=w2010, y=w2009) -> (x/y=w2008:dbl)
        "Save Data Rate (Hz)" <- w2008
        n1220 = Reciprocal(x=w2008) -> (1/x=→"Save Data Period (s)":dbl)
        n1221 = property on="Scan steps (AOD)" class="DigNum (strict)"("Val(Sgnl)"=w2006) -> ()  [unwired: 2 in, 2 out]
        n1222 = Multiply(x=w1995, y="# Samples/trap") -> (x*y=w1993:u32)
        "Counts/DMA" <- w1993
        n1223 = property on="Trap Disp. Downsample" class="DigNum (strict)"("Maximum"="# Samples/trap") -> ()  [unwired: 2 in, 2 out]
        n1224 = Multiply(x=w1998, y="# Samples/trap") -> (x*y=w1987:u32)
        "# Samples/channel" <- w1987
        n1225 = Multiply(x=w1987, y=u32 8) -> (x*y=→"Trap AI Elements/DMA read":u32)
        n1226 = local read "APD Int. Count"() -> (w1994:u32)
        n1227 = Multiply(x=w1987, y=u32 5) -> (x*y=→"Trap Pos Elements/DMA read":u32)
        n1228 = Divide(x=w1993, y=w1994) -> (x/y=w1984:dbl)
        "APD Samples/FIFO Acq." <- w1984
        n1229 = Divide(x=w1993, y=40000000.0) -> (x/y=w1991:dbl)
        "DMA Update Period (s)" <- w1991
        n1230 = local read "Number of APDs"() -> (w1977:u8)
        n1231 = Multiply(x=w1977, y=w1984) -> (x*y=→"APD Elements/DMA read":dbl)
        n1232 = property on="APD Disp. Downsample" class="DigNum (strict)"("Maximum"=w1984) -> ()  [unwired: 2 in, 2 out]
        n1233 = local read "N sets to save"() -> (w2003:u32)
        n1234 = Multiply(x=w1991, y=w2003) -> (x*y=→"Total Time (s) 2":dbl)
        "FPGA Averaging" <- FALSE ("FPGA Averaging")
      }
      event "Remove Offset": Value Change {
        n1235 = event-data() -> ()  [unwired: 7 out]
        n1236 = local write "Remove Offset"(FALSE ("Remove Offset")) -> ()
        n1237 = local read "Bead Mean (nm)"() -> (w2015:dbl)
        n1238 = local read "Offset (nm)"() -> (w2016:dbl)
        n1239 = Add(x=w2015, y=w2016) -> (x+y=w2014:dbl)
        n1240 = local write "Offset (nm)"(w2014) -> ()
      }
      event "Detector Type": Value Change {
        n1241 = event-data() -> ()  [unwired: 7 out]
        n1242 = local read "AI labels"() -> (w2020:string[])
        n1243 = property on="High Res. Display" class="Ring (strict)"("Strings []"=w2020) -> ()  [unwired: 2 in, 2 out]
        n1244 = Build Array (concatenate)(w2020, "none") -> (w2021:string[])
        n1245 = property on="FFT 1 Choice 1" class="Ring (strict)"("Strings []"=w2021) -> ()  [unwired: 2 in, 2 out]
        n1246 = property on="FFT 1 Choice 2" class="Ring (strict)"("Strings []"=w2021) -> ()  [unwired: 2 in, 2 out]
        n1247 = property on="FFT 2 Choice 1" class="Ring (strict)"("Strings []"=w2021) -> ()  [unwired: 2 in, 2 out]
        n1248 = property on="FFT 2 Choice 2" class="Ring (strict)"("Strings []"=w2021) -> ()  [unwired: 2 in, 2 out]
        n1249 = Bundle("APD 1", "APD 2", "APD 3") -> (w2024:cluster{string, string, string})  [unwired: 1 out]
        n1250 = Cluster To Array(cluster=w2024) -> (array=w2022:string[])
        n1251 = Build Array (concatenate)(w2022, w2021) -> (w2026:string[])
        n1252 = Array Size(array=w2026) -> (size(s)=w2018:i32)
        n1253 = property on="Signals to Plot" class="LstBox (strict)"("Item Names"=w2026) -> ()  [unwired: 2 in, 2 out]
        n1254 = property on="Signals to Plot" class="LstBox (strict)"("Number of Rows"=w2018) -> ()  [unwired: 2 in, 2 out]
        n1255 = property on="All Signals" class="WFChart (strict)"("LegNumRows"=w2018) -> ()  [unwired: 2 in, 2 out]
      }
      event "Adjust Scale\nto Mean": Value Change {
        n1256 = event-data() -> ()  [unwired: 7 out]
        n1257 = local read "APD rates cluster"() -> (w2029:T2)
        n1258 = Unbundle By Name(w2029) -> ("APD 1 Rate (Hz)"=w2028:dbl)
        n1259 = Multiply(x=1000.0, y="Above (kHz)") -> (x*y=w2035:dbl)
        n1260 = Multiply(x=1000.0, y="Below (kHz)") -> (x*y=w2033:dbl)
        n1261 = Add(x=w2035, y=w2028) -> (x+y=w2030:dbl)
        n1262 = Subtract(x=w2028, y=w2033) -> (x-y=w2031:dbl)
        n1263 = property on="APD Chart" class="WFChart (strict)"("YScale.Minimum"=w2031) -> ()  [unwired: 2 in, 2 out]
        n1264 = property on="APD Chart" class="WFChart (strict)"("YScale.Maximum"=w2030) -> ()  [unwired: 2 in, 2 out]
      }
      event "Phase adj. (AI1)", "+ phase (AI1)", "- phase (AI1)": Value Change {
        n1265 = event-data() -> ()  [unwired: 7 out]
        n1266 = Negate(x="Phase adj. (AI1)") -> (-x=w2047:i16)
        n1267 = Select(t=w2047, s="- phase (AI1)", f="Phase adj. (AI1)") -> (s? t:f=w2046:i16)
        n1268 = xnode "Read/Write Control"("FPGA VI Reference In"=w2039, "Phase count adjustment"=w2046) -> ("FPGA VI Reference Out"=w2045:T50, "error out"=w2044:errorcluster)  [unwired: 2 in]
        n1269 = Or(x="- phase (AI1)", y="+ phase (AI1)") -> (x .or. y?=w2041:bool)
        n1270 = xnode "Read/Write Control"("FPGA VI Reference In"=w2045, "error in"=w2044, "+ phase"=w2041) -> ("error out"=w2040:errorcluster)  [unwired: 1 in, 1 out]
      }
      event "Signals to Plot": Double Click {
        w2059 = u32 9868950 ("Color Box")
        n1271 = event-data() -> ("Row"=w2050:i32)  [unwired: 9 out]
        n1272 = property on="All Signals" class="WFChart (strict)"("Active Plot"=w2050) -> (error out=w2049:errorcluster)  [unwired: 2 in, 1 out]
        n1273 = property on="All Signals" class="WFChart (strict)" props=["Plot", "Plot Color", "Plot", "Visible?"](error in=w2049) -> (error out=w2052:errorcluster, "Plot.Visible?"=w2051:bool)  [unwired: 1 in, 2 out]
        n1274 = Select(t=FALSE ("Plot.Visible"), s=w2051, f=TRUE ("Plot.Visible")) -> (s? t:f=w2054:bool)
        n1275 = property on="All Signals" class="WFChart (strict)"(error in=w2052, "Plot.Visible?"=w2054) -> (error out=w2053:errorcluster)  [unwired: 1 in, 1 out]
        n1276 = property on="All Signals" class="WFChart (strict)"(error in=w2053) -> (error out=w2055:errorcluster, "Plot.Plot Color"=w2056:u32)  [unwired: 1 in, 1 out]
        n1277 = property on="Signals to Plot" class="LstBox (strict)"(error in=w2055, "Active Row"=w2050) -> (error out=w2060:errorcluster)  [unwired: 1 in, 1 out]
        n1278 = Select(t=w2056, s=w2054, f=u32 0) -> (s? t:f=w2061:u32)
        n1279 = property on="Signals to Plot" class="LstBox (strict)"(error in=w2060, "CellFontColor"=w2061, "SelColor"=w2059, "CellBG"=w2059, "CellFontSize"=u32 20 ("Active Row:Cell Font:Size"), "CellFontBold"=TRUE ("Active Row:Cell Font:Bold")) -> ()  [unwired: 1 in, 2 out]
      }
      event "BD 1 Frequency 1 (MHz)", "BD 1 Frequency 2 (MHz)", "BD 1 Frequency 3 (MHz)", "BD 2 Frequency 1 (MHz)", "BD 2 Frequency 2 (MHz)", "BD 2 Frequency 3 (MHz)", "Trap Delta (MHz)", "Update all trap values": Value Change {
        # "This is so you can set trap frequencies\nvia local variables and then update\nall at once"
        n1280 = event-data() -> ("CtlRef"=w2069:refnum<vi>)  [unwired: 6 out]
        n1281 = control-ref of="Trap Delta (MHz)"() -> (w2068:refnum<vi>)
        n1282 = Equal?(x=w2068, y=w2069) -> (x = y?=w2067:bool)
        n1283 = local write "Update all trap values"(FALSE ("Update all trap values")) -> ()
        n1284 = case shown="False" "Oscillate Set 1" {
          tunnel: w2067 -> [w2083 _]
          tunnel: w2065 -> [w2081 _]
          frame False {
            n1285 = local read "BD 1 Frequency 2 (MHz)"() -> (w2079:dbl)
            n1286 = case shown="False" "Symmetric?" {
              tunnel: "Trap Delta (MHz)" -> [w2105 w2112]
              tunnel: [w2106 w2110] -> w2071
              tunnel: [w2104 w2107] -> w2073
              tunnel: w2079 -> [w2106 _]
              frame False {
                n1287 = Subtract(x=w2106, y=w2105) -> (x-y=w2104:dbl)
              }
              frame True {
                w2109 = 75
                n1288 = Divide(x=w2112, y=2.0) -> (x/y=w2108:dbl)
                n1289 = Add(x=w2108, y=w2109) -> (x+y=w2110:dbl)
                n1290 = Subtract(x=w2109, y=w2108) -> (x-y=w2107:dbl)
              }
            }
            n1291 = local read "BD 1 Frequency 1 (MHz)"() -> (w2074:dbl)
            n1292 = Not(x="Symmetric?") -> (.not. x?=w2077:bool)
            n1293 = And(x=w2077, y="move Con X?") -> (x .and. y?=w2075:bool)
            n1294 = Subtract(x=w2074, y=w2073) -> (x-y=w2072:dbl)
            n1295 = Select(t=w2073, s=w2083, f=w2074) -> (s? t:f=w2082:dbl)
            n1296 = local read "Y RF Frequency Limits (MHz)"() -> (w2084:T24)
            n1297 = case shown="True" w2075 {
              tunnel: w2072 -> [_ w2103]
              frame False {
              }
              frame True {
                n1298 = property on="AOM X Cal (nm/MHz)" class="DigNum (strict)"() -> ("Value"=w2102:dbl)  [unwired: 2 in, 2 out]
                n1299 = property on="MCL Step Position Ratio" class="DigNum (strict)"() -> ("Value"=w2096:dbl)  [unwired: 2 in, 2 out]
                n1300 = Compound Arithmetic op=MULTIPLY(w2103, w2102, w2096) -> (w2101:dbl)
                n1301 = property on="MCL X Cal (nm/V)" class="DigNum (strict)"() -> ("Value"=w2100:dbl)  [unwired: 2 in, 2 out]
                n1302 = Divide(x=w2101, y=w2100) -> (x/y=w2099:dbl)
                n1303 = property on="AO2" class="Slide (strict)"() -> ("Value"=w2098:dbl)  [unwired: 2 in, 2 out]
                n1304 = Add(x=w2099, y=w2098) -> (x+y=w2097:dbl)
                n1305 = property on="AO2" class="Slide (strict)"("Val(Sgnl)"=w2097) -> ()  [unwired: 2 in, 2 out]
              }
            }
            n1306 = local read "X RF Frequency Limits (MHz)"() -> (w2085:T24)
            n1307 = local write "BD 1 Frequency 1 (MHz)"(w2082) -> ()
            n1308 = local read "BD 1 Frequency 3 (MHz)"() -> (w2094:dbl)
            n1309 = local read "BD 2 Frequency 1 (MHz)"() -> (w2088:dbl)
            n1310 = local read "BD 2 Frequency 2 (MHz)"() -> (w2087:dbl)
            n1311 = local read "BD 2 Frequency 3 (MHz)"() -> (w2095:dbl)
            n1312 = call "set RF board frequency - interlace.vi"("Board 2 Frequency Limits"=w2084, "Board 1 Frequency Limits"=w2085, "FPGA VI Reference In"=w2081, "Board 2 Frequency 3 (MHz)"=w2095, "Board 1 Frequency 3 (MHz)"=w2094, "Board 2 Frequency 2 (MHz)"=w2087, "Board 2 Frequency 1 (MHz)"=w2088, "Board 1 Frequency 2 (MHz)"=w2071, "Board 1 Frequency 1  (MHz)"=w2082) -> ()  [unwired: 1 in, 2 out]
